vi "test-linear-filter-test-00.vi"() -> (3 "Passed":bool)   [LabVIEW 2019]
uses:
  <vilib>/Rock Robotics/WPI/ThirdParty/JAS_Junk/TrajLib/Trajectory_Library.lvlib
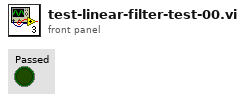
[diagram p1: front panel]
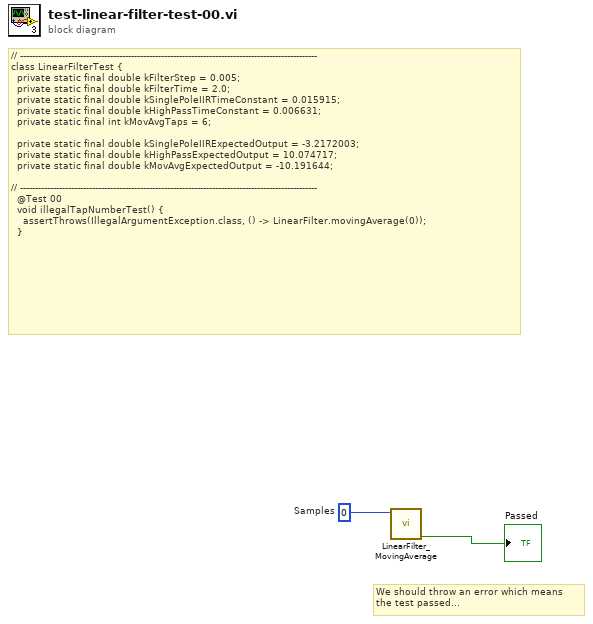
[diagram p0: block diagram]
diagram:
  w2 = 0  # Samples
  # "We should throw an error which means\nthe test passed..."
  # "// ---------------------------------------------------------------------------------------------------\nclass LinearFilterTest {\n  private static final double kFilterStep = 0.005;\n  private static final double kFilterTime = 2.0;\n  private static final double kSinglePoleIIRTimeConstant = 0.015915;\n  private static final double kHighPassTimeConstant = 0.006631;\n  private static final int kMovAvgTaps = 6;\n\n  private static final double kSinglePoleIIRExpectedOutput = -3.2172003;\n  private static final double kHighPassExpectedOutput = 10.074717;\n  private static final double kMovAvgExpectedOutput = -10.191644;\n\n// ---------------------------------------------------------------------------------------------------\n  @Test 00\n  void illegalTapNumberTest() {\n    assertThrows(IllegalArgumentException.class, () -> LinearFilter.movingAverage(0));\n  }"
  n1 = call <vilib>:"LinearFilter_MovingAverage.vi"("Samples"=w2) -> ("Error"=→"Passed":bool)  [unwired: 9 in, 1 out]
